vi "Initialize Test Device Modbus Client TCP.vi"(5 "timeout, ms (300)":u32=300, 6 "station address (255)":u8=255, 7 "protocol (TCP)":enum16{"RTU", "ASCII", "TCP"}(ring)=enum."TCP", 8 "error in (no error)":errorcluster, 9 "port (502)":u16=502, 10 "ip address":string, 11 "TD in":refnum<class "Test Device.lvclass">) -> (0 "error out":errorcluster, 3 "TD out":refnum<class "Test Device.lvclass">)   [LabVIEW 2015, in "Test Device.lvclass"]
uses:
  Test Device.lvclass
  <vilib>/plasmapper/PL BlackBox Modbus CLient/PL BlackBox Modbus Client.lvclass
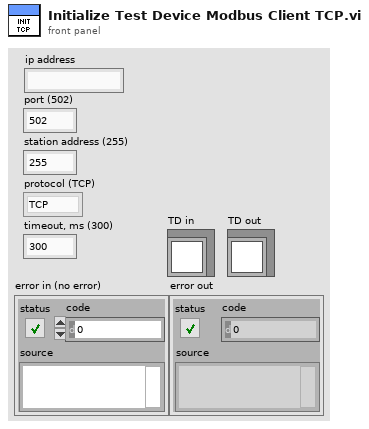
[diagram p1: front panel]
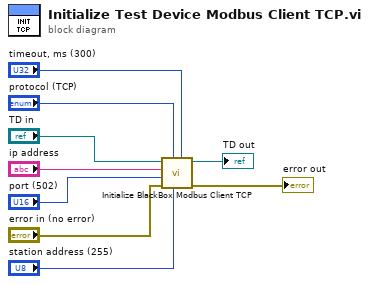
[diagram p0: block diagram]
diagram:
  n1 = call <vilib>:"Initialize BlackBox Modbus Client TCP.vi"("timeout, ms (300)"="timeout, ms (300)", "station address (255)"="station address (255)", "protocol (TCP)"="protocol (TCP)", "error in (no error)"="error in (no error)", "port (502)"="port (502)", "ip address"="ip address", "PLBB in"="TD in") -> ("error out"=→"error out":errorcluster, "PLBB out"=→"TD out":refnum<class "Test Device.lvclass">)  [unwired: 3 in]
